vi "sub_Write Error Log.vi"(8 "error in (no error)":errorcluster, 9 "Data":variant) -> (0 "error out":errorcluster)   [LabVIEW 2016, in "System.lvlib"]
uses:
  System.lvlib
  Controls/Control_Error Data.ctl
  <vilib>/Utility/error.llb/DialogType.ctl
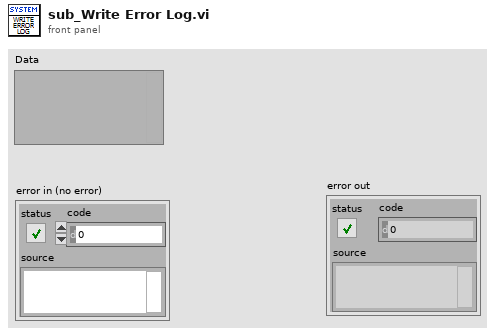
[diagram p1: front panel]
types:
  T1 = typedef "System.lvlib/Control_Error Data.ctl" = cluster{"Time":timestamp, "Error":errorcluster}
  T2 = typedef "DialogType.ctl" = u16
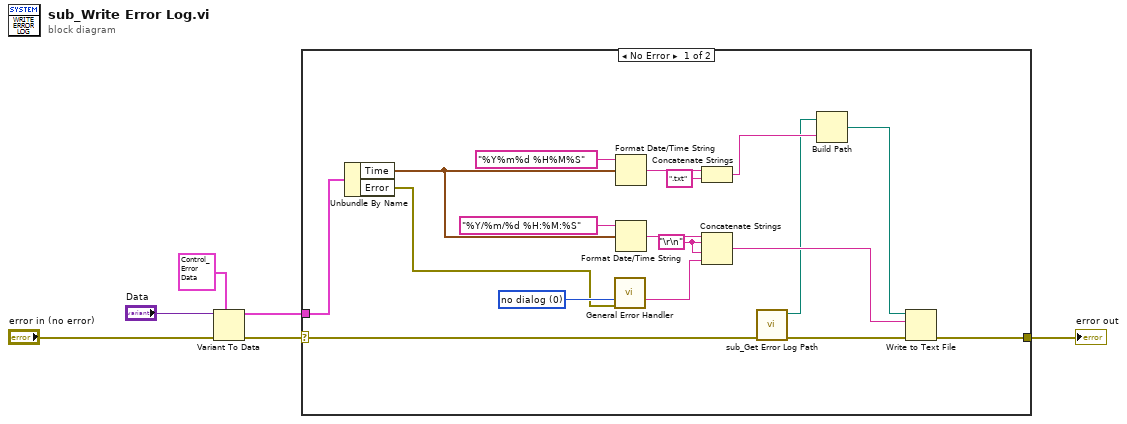
[diagram p0: block diagram]
diagram:
  n1 = Variant To Data(error in="error in (no error)", type=T1 {"Time"=timestamp(0 s since 1904-01-01), "Error"={"status"=FALSE, "code"=0, "source"=""}} ("Error Data"), Variant="Data") -> (data=w4:T1, error out=w5:errorcluster)
  n2 = case shown="No Error" w5 {
    selector: w5 -> [w9 _]
    tunnel: w4 -> [w24 _]
    tunnel: [w12 _] -> w2
    frame No Error {
      w10 = "\r\n"
      w18 = T2 0 items=["no dialog", "OK message", "continue or stop message", "OK message + warnings", "continue/stop + warnings"] ("type of dialog (OK msg:1)")
      n3 = Unbundle By Name(w24) -> ("Time"=w19:timestamp, "Error"=w17:errorcluster)
      n4 = call <vilib>:"General Error Handler.vi"("type of dialog (OK msg:1)"=w18, "error in (no error)"=w17) -> ("message"=w15:string)  [unwired: 9 in, 4 out]
      n5 = Format Date/Time String(time format string (%c)="%Y%m%d %H%M%S", seconds (now)=w19) -> (date/time string=w22:string)  [unwired: 1 in]
      n6 = Format Date/Time String(time format string (%c)="%Y/%m/%d %H:%M:%S", seconds (now)=w19) -> (date/time string=w16:string)  [unwired: 1 in]
      n7 = Concatenate Strings(w22, ".txt" ("string")) -> (w14:string)
      n8 = Concatenate Strings(w16, w10, w10, w15) -> (w13:string)
      n9 = call "sub_Get Error Log Path.vi"("error in (no error)"=w9) -> ("error out"=w8:errorcluster, "Path"=w7:path)  [unwired: 9 in]
      n10 = Build Path(base path=w7, name or relative path=w14) -> (appended path=w11:path)
      n11 = Write to Text File(file (use dialog)=w11, text=w13, error in=w8) -> (error out=w12:errorcluster)  [unwired: 1 in, 2 out]
    }
    frame Error {
    }
  }
  "error out" <- w2
